vi "_TangoExecuteCommand.vi"(2 "error in":errorcluster, 3 "argin":cluster{"num data":u8[], "str data":string[]}, 4 "command name":string, 5 "device name":string) -> (0 "error out":errorcluster, 1 "argout":cluster{"num data":u8[], "str data":string[]})   [LabVIEW 2014, in "tango.lvlib"]
uses:
  tango.lvlib
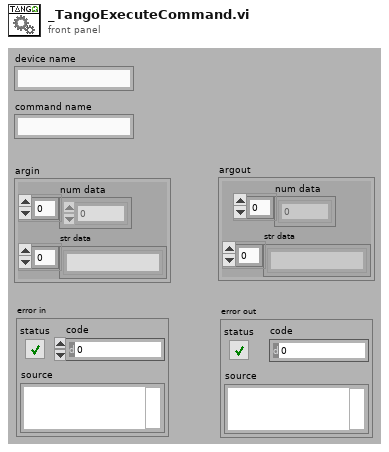
[diagram p1: front panel]
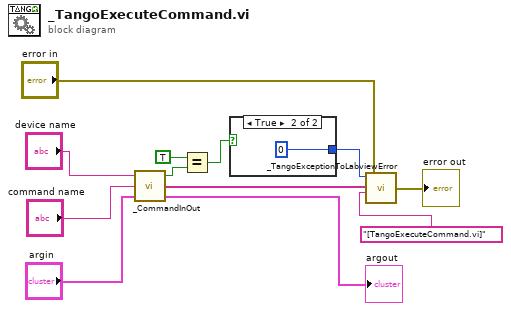
[diagram p0: block diagram]
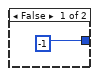
[diagram p2: hidden frame]
diagram:
  n1 = call "_CommandInOut.vi"("argin"="argin", "command name"="command name", "device name"="device name") -> ("argout"=→"argout":cluster{"num data":u8[], "str data":string[]}, "error stack"=w1:string[], "success"=w5:bool)
  n2 = Equal?(x=TRUE, y=w5) -> (x = y?=w3:bool)
  n3 = case shown="True" w3 {
    tunnel: [-1 0] -> w2
    frame False {
    }
    frame True {
    }
  }
  n4 = call "_TangoExceptionToLabviewError.vi"("error in"="error in", "location"="[TangoExecuteCommand.vi]", "error stack"=w1, "error code"=w2) -> ("error out"=→"error out":errorcluster)
